vi "Save Data to Database.vi"(7 "Database Connection":refnum<k7>, 8 "Error In":errorcluster, 10 "Data (EU)":dbl[](array[numeric]) format="%.2g", 11 "Channel Settings":T1(array[cluster]) {"Vmax" min=-10.0 max=10.0 step=1.0; "Vmin" min=-10.0 max=10.0 step=1.0}) -> (0 "Error Out":errorcluster)   [LabVIEW 2018]
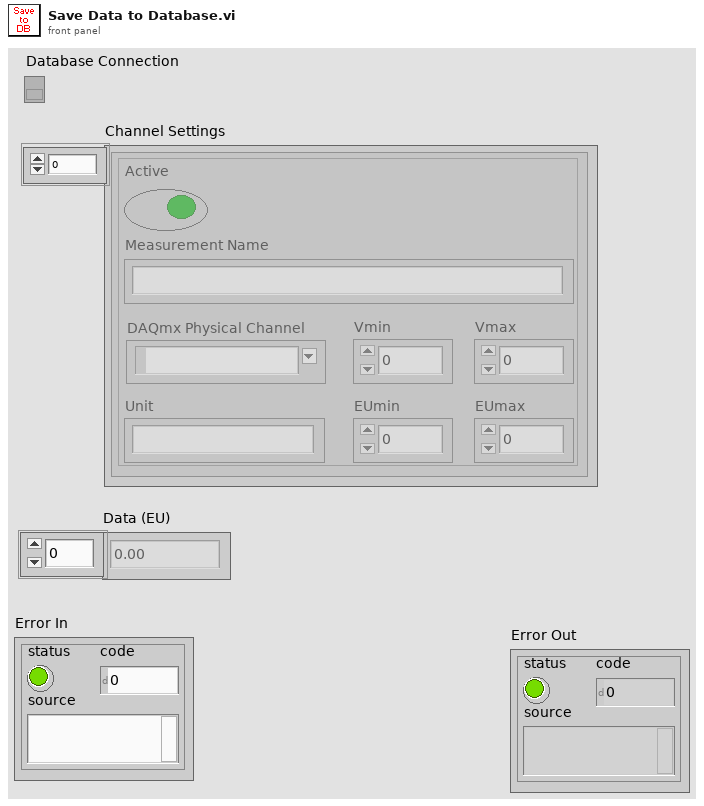
[diagram p1: front panel]
types:
  T1 = cluster{"Active":bool, "Measurement Name":string, "DAQmx Physical Channel":tag, "Vmin":dbl, "Vmax":dbl, "Unit":string, "EUmin":dbl, "EUmax":dbl}[]
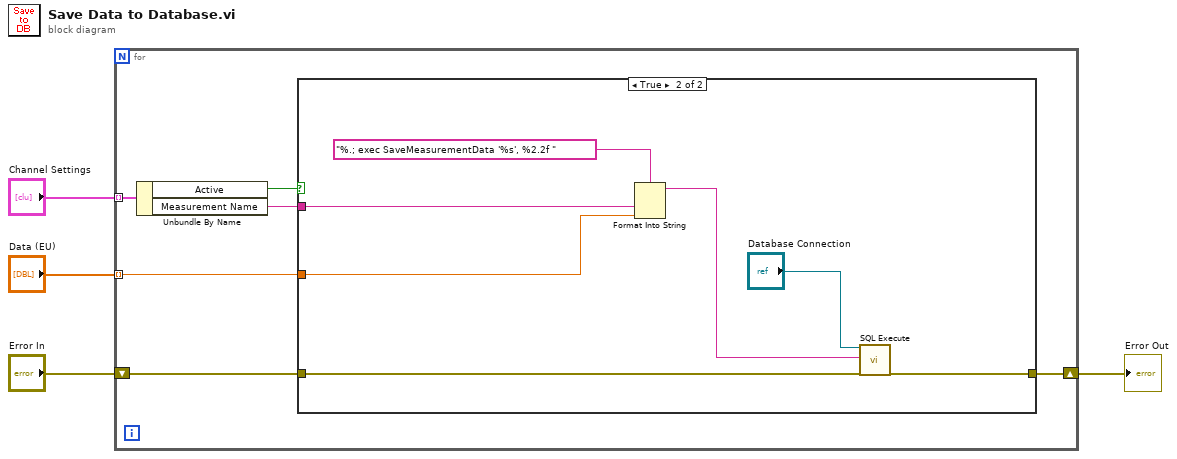
[diagram p0: block diagram]
diagram:
  n1 = for {
    tunnel: "Data (EU)" -> [w8] mode=indexing
    shift-right: [w9] -> w4
    shift-left: "Error In" -> [w10]
    tunnel: "Channel Settings" -> [w7] mode=indexing
    n2 = Unbundle By Name(w7) -> ("Active"=w6:bool, "Measurement Name"=w5:string)
    n3 = case shown="True" w6 {
      tunnel: w10 -> [w11 w16]
      tunnel: [w11 w15] -> w9
      tunnel: w8 -> [_ w13]
      tunnel: w5 -> [_ w12]
      frame False {
      }
      frame True {
        n4 = Format Into String "Format Into String"(format string="%.; exec SaveMeasurementData '%s', %2.2f ", w12, w13) -> (resulting string=w17:string)  [unwired: 2 in, 1 out]
        n5 = call <vilib>:"SQL Execute.vi"("Connection In"="Database Connection", "SQL Query"=w17, "Error in (no error)"=w16) -> ("Error out"=w15:errorcluster)  [unwired: 15 in, 1 out]
      }
    }
  }
  "Error Out" <- w4
